vi "IEEE754 V1.1.vi"(10 "低位16":i16 format="%04x", 11 "高位16":i16=17244 format="%04x") -> (3 "输出浮点型":dbl)   [LabVIEW 2015]
panel:
  out "HexFormat":i32=1130102784 format="%x"
  # "IEEE754 2个16位整型转换为浮点型"
  # "输出"
  # "输入"
  # "1、程序将两个16位整型转换为一个32为的浮点型数据，转换原则按照IEEE754标准进行；\n2、高16、低16位和合并后的Hex格式数据都是16进制显示；\n3、输出浮点型是转换后的数据。"
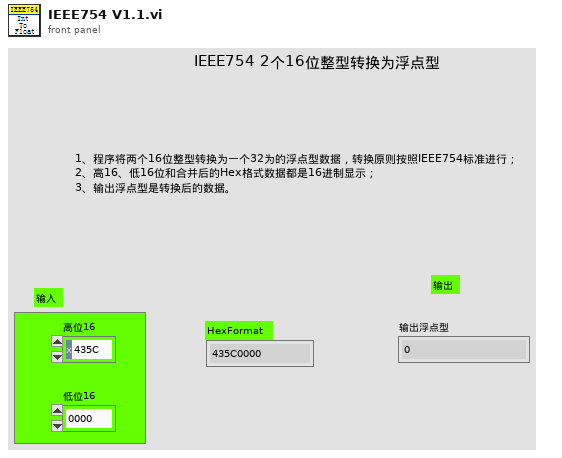
[diagram p1: front panel]
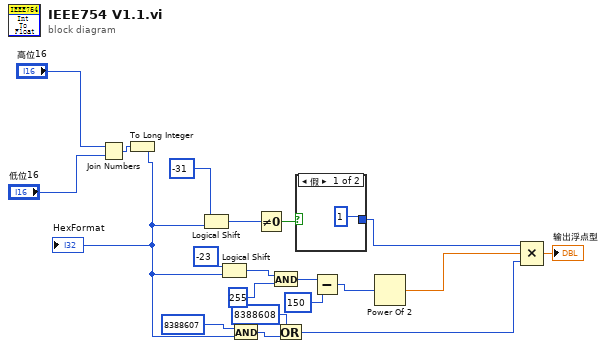
[diagram p0: block diagram]
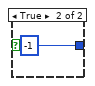
[diagram p2: hidden frame]
diagram:
  n1 = Join Numbers(hi="高位16", lo="低位16") -> ((hi.lo)=w2:u32)
  n2 = To Long Integer(number=w2) -> (32bit integer=w1:i32)
  "HexFormat" <- w1
  n3 = Logical Shift(y=-31, x=w1) -> (x << y=w19:i32)
  n4 = Logical Shift(y=-23, x=w1) -> (x << y=w16:i32)
  n5 = And(x=8388607, y=w1) -> (x .and. y?=w11:i32)
  n6 = Not Equal To 0?(x=w19) -> (x != 0?=w18:bool)
  n7 = And(x=w16, y=255) -> (x .and. y?=w14:i32)
  n8 = Or(x=8388608, y=w11) -> (x .or. y?=w8:i32)
  n9 = case shown="假" w18 {
    tunnel: [1 -1] -> w9
    frame False {
    }
    frame True {
    }
  }
  n10 = Subtract(x=w14, y=150) -> (x-y=w6:i32)
  n11 = Power Of 2(x=w6) -> (2^x=w5:dbl)
  n12 = Compound Arithmetic op=MULTIPLY(w9, w5, w8) -> (→"输出浮点型":dbl)
